vi "CreateResultTreeListener.vi"(8 "error in (no error)":errorcluster, 10 "ResultTree":refnum<class "ResultTree.lvclass">) -> (0 "error out":errorcluster, 3 "ResultTreeListener out":refnum<class "ResultTreeListener.lvclass">)   [LabVIEW 2017, in "ResultTreeListener.lvclass"]
doc: "Creates a new listener for a <B>ResultTree</B> object."
uses:
  ResultTreeListener.lvclass
  ResultTree/ResultTree.lvclass
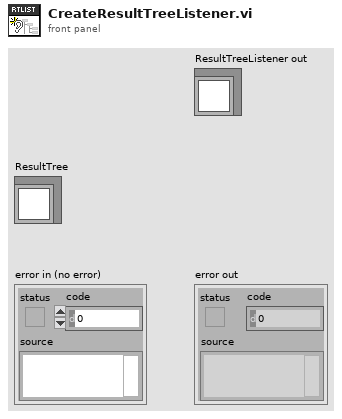
[diagram p1: front panel]
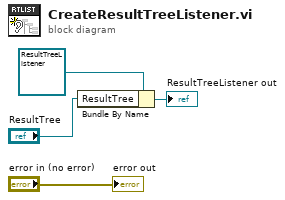
[diagram p0: block diagram]
diagram:
  n1 = Bundle By Name(cluster=refnum<class "ResultTreeListener.lvclass"> refnum ("ResultTreeListener in"), "ResultTree"="ResultTree") -> (→"ResultTreeListener out":refnum<class "ResultTreeListener.lvclass">)
  "error out" <- "error in (no error)"
